vi "1553B_帧解析_字符串_v4_27.vi"(11 "输入簇":T1) -> (2 "脉冲数":string, 3 "温度":string)   [LabVIEW 2012]
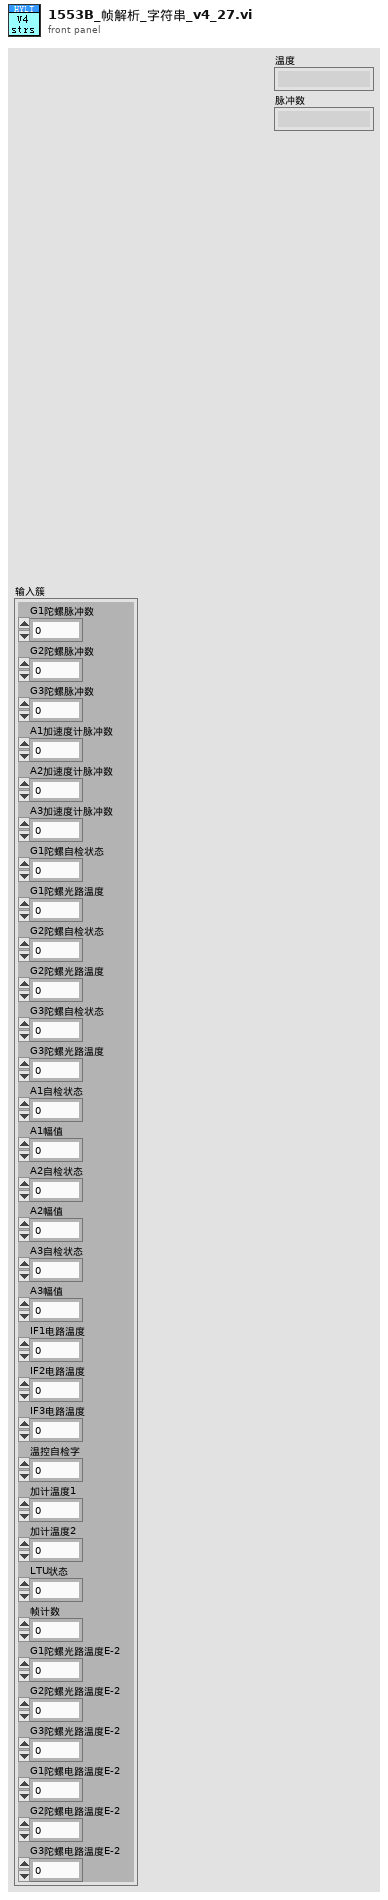
[diagram p1: front panel]
types:
  T1 = cluster{"G1陀螺脉冲数":i32, "G2陀螺脉冲数":i32, "G3陀螺脉冲数":i32, "A1加速度计脉冲数":i16, "A2加速度计脉冲数":i16, "A3加速度计脉冲数":i16, "G1陀螺自检状态":u8, "G1陀螺光路温度":i8, "G2陀螺自检状态":u8, "G2陀螺光路温度":i8, "G3陀螺自检状态":u8, "G3陀螺光路温度":i8, "A1自检状态":u8, "A1幅值":u8, "A2自检状态":u8, "A2幅值":u8, "A3自检状态":u8, "A3幅值":u8, "IF1电路温度":i8, "IF2电路温度":i8, "IF3电路温度":i8, "温控自检字":u8, "加计温度1":i16, "加计温度2":i16, "LTU状态":u8, "帧计数":u8, "G1陀螺光路温度E-2":i16, "G2陀螺光路温度E-2":i16, "G3陀螺光路温度E-2":i16, "G1陀螺电路温度E-2":i16, "G2陀螺电路温度E-2":i16, "G3陀螺电路温度E-2":i16}
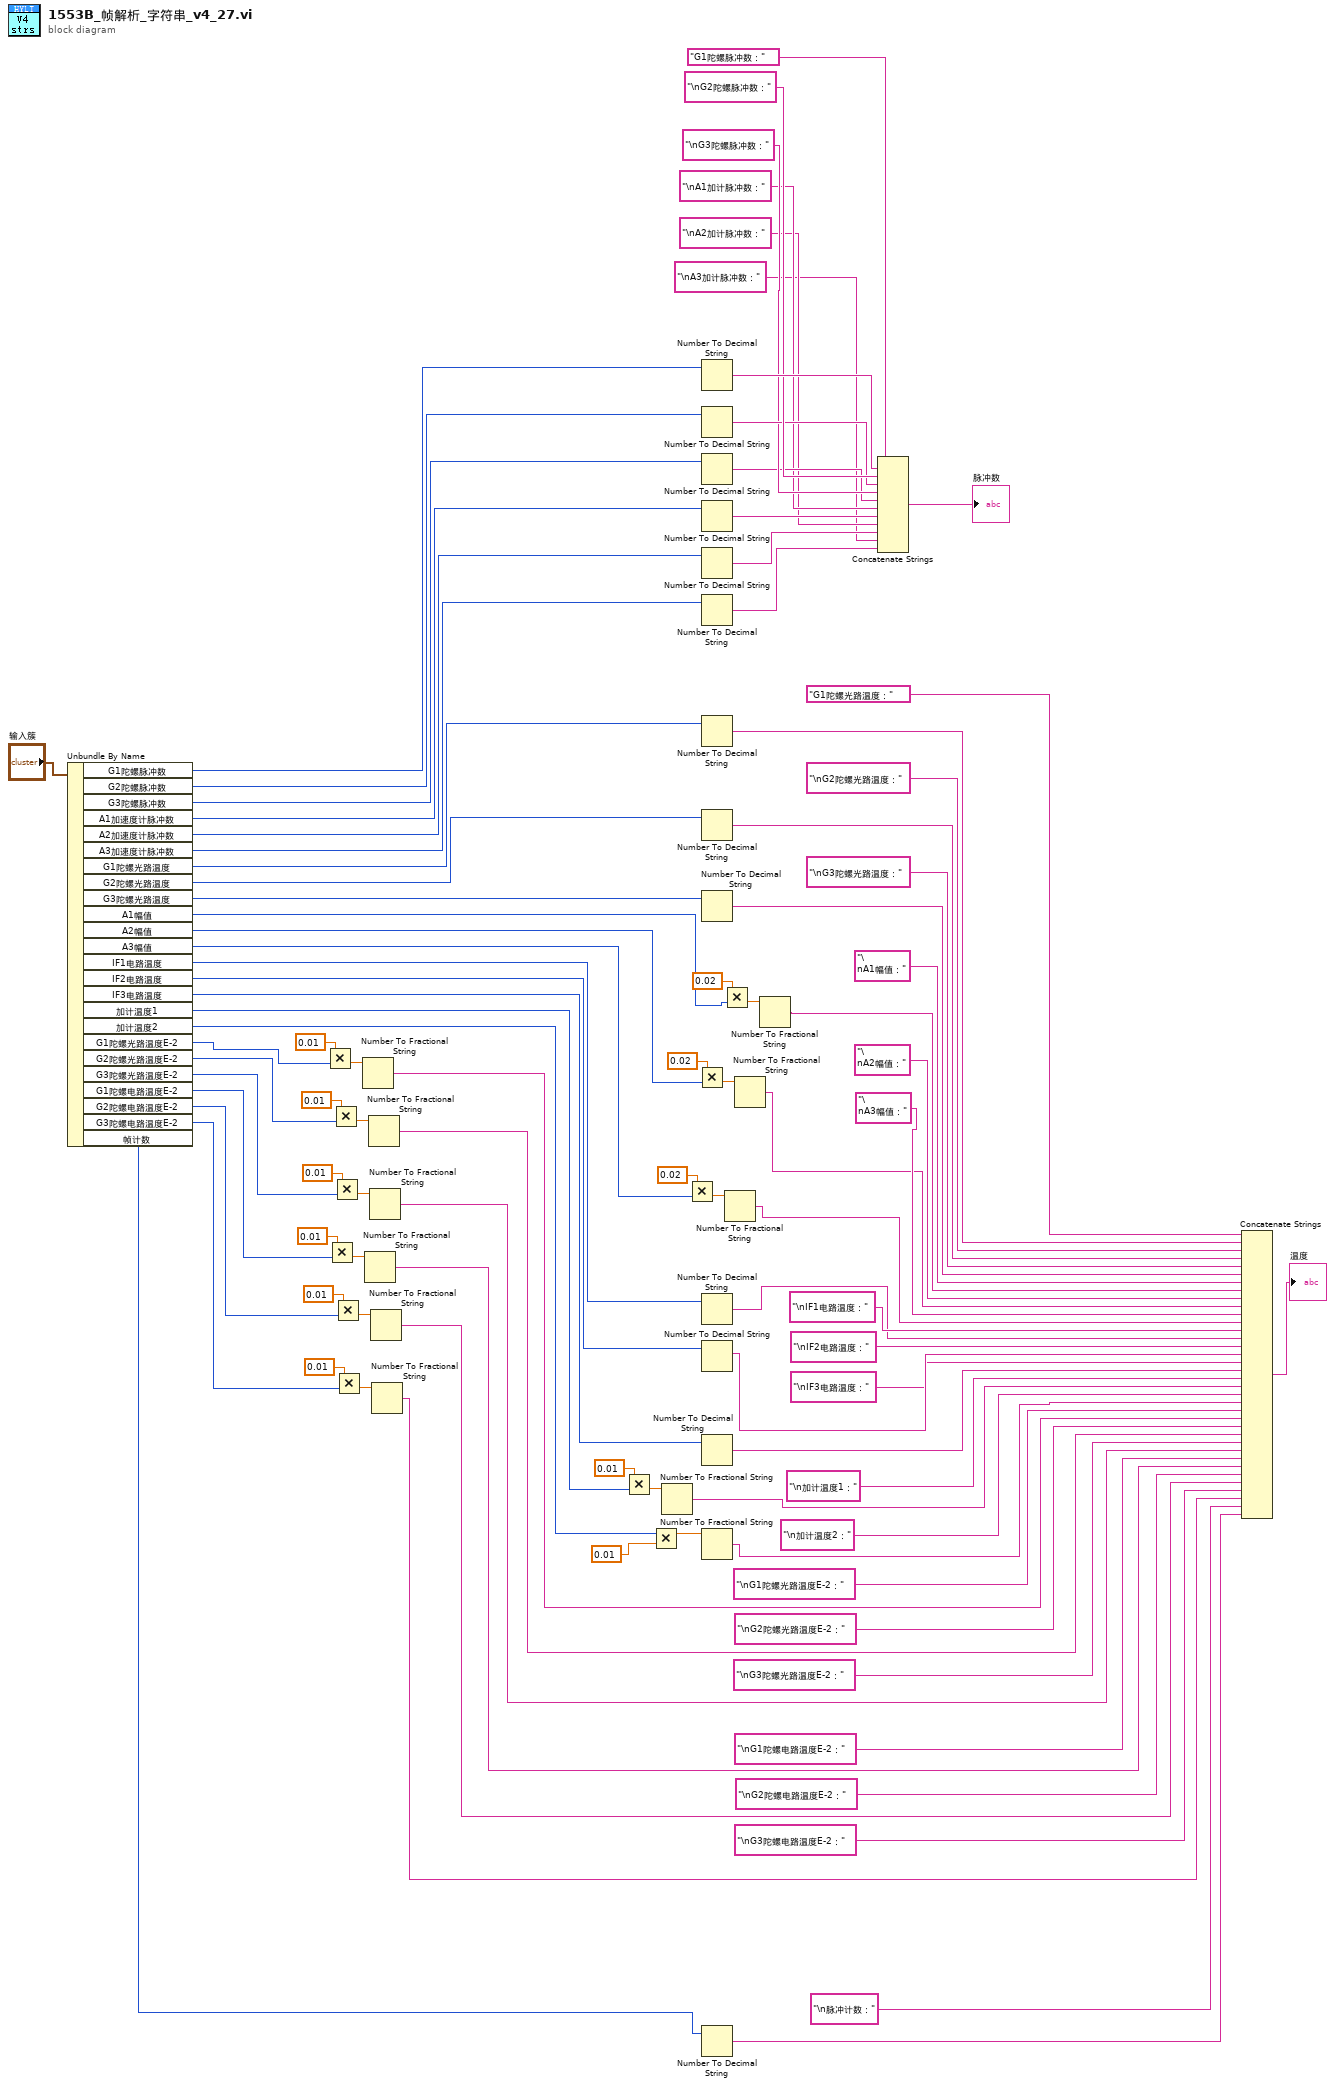
[diagram p0: block diagram]
diagram:
  n1 = Unbundle By Name("输入簇") -> ("G1陀螺脉冲数"=w83:i32, "G2陀螺脉冲数"=w82:i32, "G3陀螺脉冲数"=w81:i32, "A1加速度计脉冲数"=w80:i16, "A2加速度计脉冲数"=w97:i16, "A3加速度计脉冲数"=w96:i16, "G1陀螺光路温度"=w71:i8, "G2陀螺光路温度"=w70:i8, "G3陀螺光路温度"=w69:i8, "A1幅值"=w35:u8, "A2幅值"=w31:u8, "A3幅值"=w34:u8, "IF1电路温度"=w66:i8, "IF2电路温度"=w65:i8, "IF3电路温度"=w64:i8, "加计温度1"=w55:i16, "加计温度2"=w54:i16, "G1陀螺光路温度E-2"=w24:i16, "G2陀螺光路温度E-2"=w23:i16, "G3陀螺光路温度E-2"=w22:i16, "G1陀螺电路温度E-2"=w15:i16, "G2陀螺电路温度E-2"=w14:i16, "G3陀螺电路温度E-2"=w13:i16, "帧计数"=w50:u8)
  n2 = Multiply(x=0.01, y=w24) -> (x*y=w30:dbl)
  n3 = Multiply(x=0.01, y=w15) -> (x*y=w16:dbl)
  n4 = Multiply(x=0.01, y=w23) -> (x*y=w27:dbl)
  n5 = Multiply(x=0.01, y=w22) -> (x*y=w26:dbl)
  n6 = Multiply(x=0.01, y=w14) -> (x*y=w19:dbl)
  n7 = Multiply(x=0.01, y=w13) -> (x*y=w20:dbl)
  n8 = Number To Fractional String(number=w30) -> (F-format string=w6:string)  [unwired: 3 in]
  n9 = Number To Fractional String(number=w16) -> (F-format string=w3:string)  [unwired: 3 in]
  n10 = Number To Fractional String(number=w27) -> (F-format string=w5:string)  [unwired: 3 in]
  n11 = Number To Fractional String(number=w26) -> (F-format string=w4:string)  [unwired: 3 in]
  n12 = Number To Fractional String(number=w19) -> (F-format string=w2:string)  [unwired: 3 in]
  n13 = Number To Fractional String(number=w20) -> (F-format string=w1:string)  [unwired: 3 in]
  n14 = Multiply(x=0.01, y=w55) -> (x*y=w46:dbl)
  n15 = Multiply(x=w54, y=0.01) -> (x*y=w44:dbl)
  n16 = Number To Fractional String(number=w46) -> (F-format string=w45:string)  [unwired: 3 in]
  n17 = Multiply(x=0.02, y=w34) -> (x*y=w41:dbl)
  n18 = Multiply(x=0.02, y=w31) -> (x*y=w39:dbl)
  n19 = Number To Decimal String(number=w83) -> (decimal integer string=w94:string)  [unwired: 1 in]
  n20 = Number To Decimal String(number=w82) -> (decimal integer string=w92:string)  [unwired: 1 in]
  n21 = Number To Decimal String(number=w81) -> (decimal integer string=w90:string)  [unwired: 1 in]
  n22 = Number To Decimal String(number=w80) -> (decimal integer string=w88:string)  [unwired: 1 in]
  n23 = Number To Decimal String(number=w97) -> (decimal integer string=w86:string)  [unwired: 1 in]
  n24 = Number To Decimal String(number=w96) -> (decimal integer string=w84:string)  [unwired: 1 in]
  n25 = Number To Decimal String(number=w71) -> (decimal integer string=w73:string)  [unwired: 1 in]
  n26 = Number To Decimal String(number=w70) -> (decimal integer string=w75:string)  [unwired: 1 in]
  n27 = Number To Decimal String(number=w69) -> (decimal integer string=w77:string)  [unwired: 1 in]
  n28 = Number To Decimal String(number=w66) -> (decimal integer string=w60:string)  [unwired: 1 in]
  n29 = Number To Decimal String(number=w65) -> (decimal integer string=w58:string)  [unwired: 1 in]
  n30 = Number To Decimal String(number=w64) -> (decimal integer string=w56:string)  [unwired: 1 in]
  n31 = Number To Fractional String(number=w44) -> (F-format string=w51:string)  [unwired: 3 in]
  n32 = Number To Decimal String(number=w50) -> (decimal integer string=w49:string)  [unwired: 1 in]
  n33 = Multiply(x=0.02, y=w35) -> (x*y=w37:dbl)
  n34 = Number To Fractional String(number=w41) -> (F-format string=w33:string)  [unwired: 3 in]
  n35 = Number To Fractional String(number=w39) -> (F-format string=w32:string)  [unwired: 3 in]
  n36 = Number To Fractional String(number=w37) -> (F-format string=w36:string)  [unwired: 3 in]
  n37 = Concatenate Strings("G1陀螺脉冲数：" ("字符串"), w94, "\nG2陀螺脉冲数：" ("字符串"), w92, "\nG3陀螺脉冲数：" ("字符串"), w90, "\nA1加计脉冲数：" ("字符串"), w88, "\nA2加计脉冲数：" ("字符串"), w86, "\nA3加计脉冲数：" ("字符串"), w84) -> (→"脉冲数":string)
  n38 = Concatenate Strings("G1陀螺光路温度：" ("字符串"), w73, "\nG2陀螺光路温度：" ("字符串"), w75, "\nG3陀螺光路温度：" ("字符串"), w77, "\nA1幅值：" ("字符串"), w36, "\nA2幅值：" ("字符串"), w32, "\nA3幅值：" ("字符串"), w33, "\nIF1电路温度：" ("字符串"), w60, "\nIF2电路温度：" ("字符串"), w58, "\nIF3电路温度：" ("字符串"), w56, "\n加计温度1：" ("字符串"), w45, "\n加计温度2：" ("字符串"), w51, "\nG1陀螺光路温度E-2：" ("字符串"), w6, "\nG2陀螺光路温度E-2：" ("字符串"), w5, "\nG3陀螺光路温度E-2：" ("字符串"), w4, "\nG1陀螺电路温度E-2：" ("字符串"), w3, "\nG2陀螺电路温度E-2：" ("字符串"), w2, "\nG3陀螺电路温度E-2：" ("字符串"), w1, "\n脉冲计数：" ("字符串"), w49) -> (→"温度":string)
